vi "Transmit CAN Test.vi"() -> ()   [LabVIEW 2015]
uses:
  <vilib>/RioEmbeddedCAN/RioEmbeddedCAN.llb/CANFrameControl.ctl
  <vilib>/RioEmbeddedCAN/RioEmbeddedCAN.llb/CANWaitInterfaceCommunicating.vi
  <vilib>/RioEmbeddedCAN/RioEmbeddedCAN.llb/CANWaitTransmitComplete.vi
  <resource>/objmgr/RioEmbeddedCANInterface.rc
panel:
  out "error out":errorcluster
  out "Baud":u32
  out "Receive Error Counter":u8
  out "Communication State":u32(ring) items=["Error Active", "Error Passive", "Bus Off", "Init"]
  out "Transmit Error Counter":u8
  in  "stop":bool
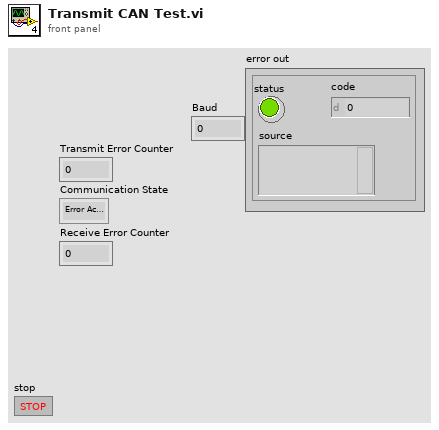
[diagram p1: front panel]
types:
  T1 = typedef "CANFrameControl.ctl" = cluster{"identifier":u32, "extended?":bool, "type":u8, "payload":u8[]}
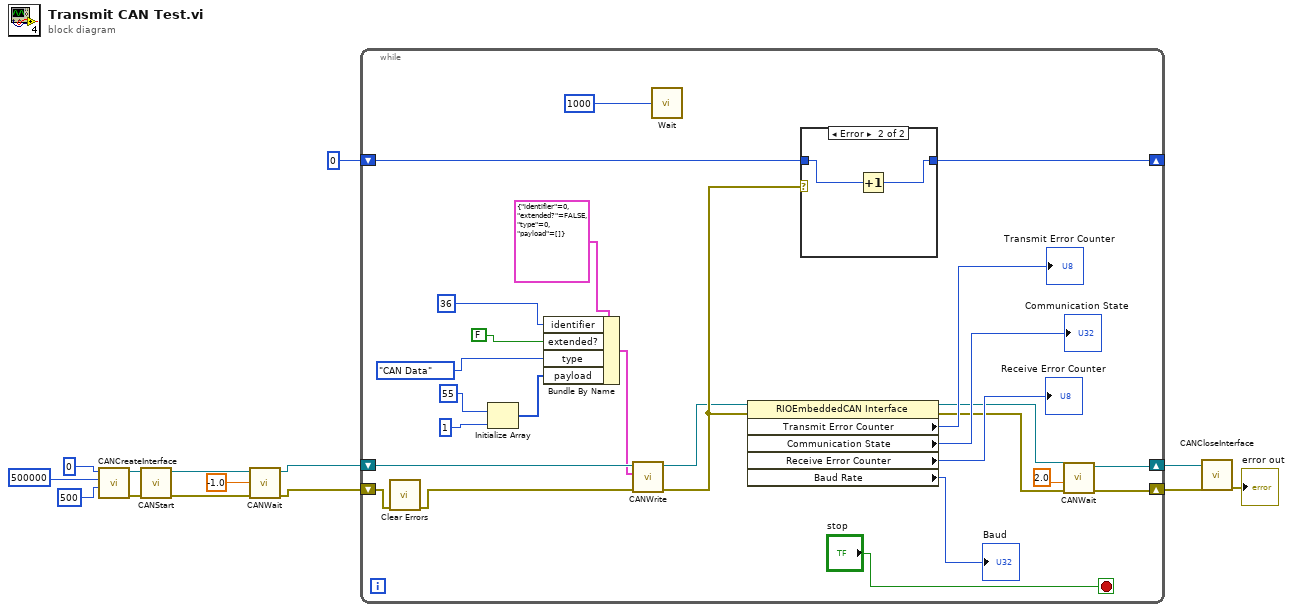
[diagram p0: block diagram]
diagram:
  n1 = call <vilib>:"CANCreateInterface.vi"("receive queue size (5)"=u32 500, "baud rate (125000 bps)"=u32 500000 ("Baud Rate"), "interface index"=u32 0) -> ("error out"=w13:errorcluster, "interface object out"=w12:refnum<k20>)  [unwired: 7 in]
  n2 = call <vilib>:"CANStart.vi"("error in (no error)"=w13, "interface object in"=w12) -> ("error out"=w4:errorcluster, "interface object out"=w6:refnum<k20>)  [unwired: 8 in]
  n3 = call-poly <vilib>:"CANWait.vi"("error in (no error)"=w4, "timeout (0 s)"=-1.0, "interface object in"=w6) -> ("error out"=w8:errorcluster, "interface object out"=w7:refnum<k20>)  [unwired: 7 in]
  n4 = while {
    shift-right: [w22] -> w3
    shift-left: w7 -> [w32]
    shift-right: [w29] -> _
    shift-left: 0 -> [w30]
    shift-right: [w21] -> w2
    shift-left: w8 -> [w18]
    stop <- "stop" stop-if-true
    n5 = call <vilib>:"Clear Errors.vi"("error in (no error)"=w18) -> ("error out"=w17:errorcluster)  [unwired: 5 in, 1 out]
    n6 = Initialize Array(u8 55, 1) -> (w34:u8[])
    n7 = Bundle By Name(cluster=T1 {"identifier"=0, "extended?"=FALSE, "type"=0, "payload"=[]} ("CAN frame"), "identifier"=u32 36, "extended?"=FALSE, "type"=enum8{"CAN Data", "CAN Remote"}."CAN Data", "payload"=w34) -> (w15:T1)
    n8 = call <vilib>:"CANWrite.vi"("error in (no error)"=w17, "CAN frame"=w15, "interface object in"=w32) -> ("error out"=w28:errorcluster, "interface object out"=w27:refnum<k20>)  [unwired: 7 in]
    n9 = call "Wait"("Count(mSec)"=1000) -> ()  [unwired: 1 out]
    n10 = property class="RIOEmbeddedCAN Interface"(reference=w27, error in=w28) -> (reference out=w23:refnum<k20>, error out=w19:errorcluster, "Transmit Error Counter"=→"Transmit Error Counter":u8, "Communication State"=→"Communication State":u32, "Receive Error Counter"=→"Receive Error Counter":u8, "Baud Rate"=→"Baud":u32)
    n11 = case shown="Error" w28 {
      tunnel: w30 -> [w41 w43]
      tunnel: [w41 w42] -> w29
      frame No Error {
      }
      frame Error {
        n12 = Increment(x=w43) -> (x+1=w42:i32)
      }
    }
    n13 = call-poly <vilib>:"CANWait.vi"("error in (no error)"=w19, "timeout (0 s)"=2.0, "interface object in"=w23) -> ("error out"=w21:errorcluster, "interface object out"=w22:refnum<k20>)  [unwired: 7 in]
  }
  n14 = call <vilib>:"CANCloseInterface.vi"("error in (no error)"=w2, "interface object in"=w3) -> ("error out"=→"error out":errorcluster)  [unwired: 9 in]
